vi "FocusLock_Ref_HX.vi"(7 "Action":enum16{"READ", "WRITE"}(ring), 10 "FocusLock Ref In":refnum<vi>) -> (2 "FocusLock Ref Out":refnum<vi>)   [LabVIEW 2014]
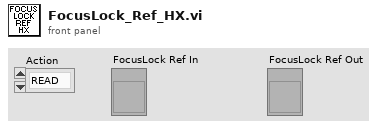
[diagram p1: front panel]
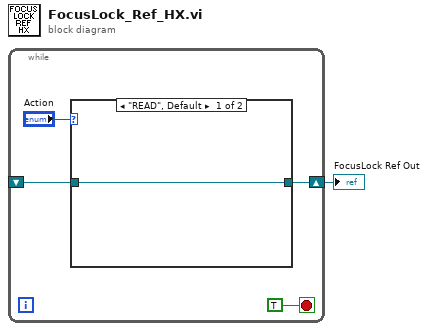
[diagram p0: block diagram]
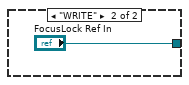
[diagram p2: hidden frame]
diagram:
  n1 = while {
    shift-right: [w3] -> w1
    shift-left: _ -> [w2]
    stop <- TRUE stop-if-true
    n2 = case shown="\"READ\", Default" "Action" {
      tunnel: [w6 "FocusLock Ref In"] -> w3
      tunnel: w2 -> [w6 _]
      frame "READ", Default {
      }
      frame "WRITE" {
      }
    }
  }
  "FocusLock Ref Out" <- w1
